vi "SIM BDF Is Jacobian Fresh.vi"(4 "BDF data out":T1, 5 "Timestep Index":dbl) -> (1 "Old Jacobian?":bool)   [LabVIEW 2020]
uses:
  SIM BDF data.ctl
  SIM Factored Matrix.ctl
  SIM BDF stages.ctl
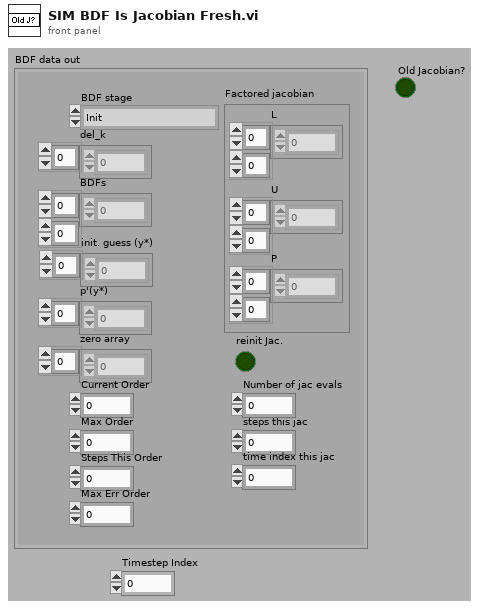
[diagram p1: front panel]
types:
  T1 = typedef "SIM BDF data.ctl" = cluster{"BDFs":dbl[][], "init. guess (y*)":dbl[], "p'(y*)":dbl[], "Factored jacobian":T2, "zero array":dbl[], "reinit Jac.":bool, "BDF stage":T3, "steps this jac":i32, "time index this jac":i32, "Number of jac evals":i32, "del_k":dbl[], "Current Order":i32, "Max Order":i32, "Steps This Order":i32, "Max Err Order":i32}
  T2 = typedef "SIM Factored Matrix.ctl" = cluster{"L":dbl[][], "U":dbl[][], "P":i32[][]}
  T3 = typedef "SIM BDF stages.ctl" = enum16{"Init", "Initial Guess", "Compute Jacobian", "Newton Iteration", "Eval Error", "Choose StepSize", "Reset BDFs"}
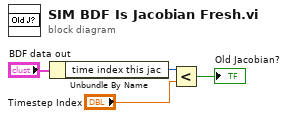
[diagram p0: block diagram]
diagram:
  n1 = Unbundle By Name("BDF data out") -> ("time index this jac"=w3:i32)
  n2 = Less?(x=w3, y="Timestep Index") -> (x < y?=→"Old Jacobian?":bool)
